vi "Test SLL DVR API Generator.vi"(6 "DVR API Suffix":string=" API", 8 "error in (no error)":errorcluster, 9 "DVR API Directory Path":path=path "D:/GitHub/LabVIEW/SLL/Tools/Class DVR API Generator/Example/APIs", 10 "Class Method Directory":path=path "D:/GitHub/LabVIEW/SLL/Tools/Class DVR API Generator/Example/Methods", 11 "Class Path":path=path "D:/GitHub/LabVIEW/SLL/Tools/Class DVR API Generator/Example/My Sample Class.lvclass") -> (0 "error out":errorcluster)   [LabVIEW 2016, in "SLL Scripting.lvlib"]
uses:
  SLL Scripting.lvlib
  SLL Class DVR API Generator.lvlib
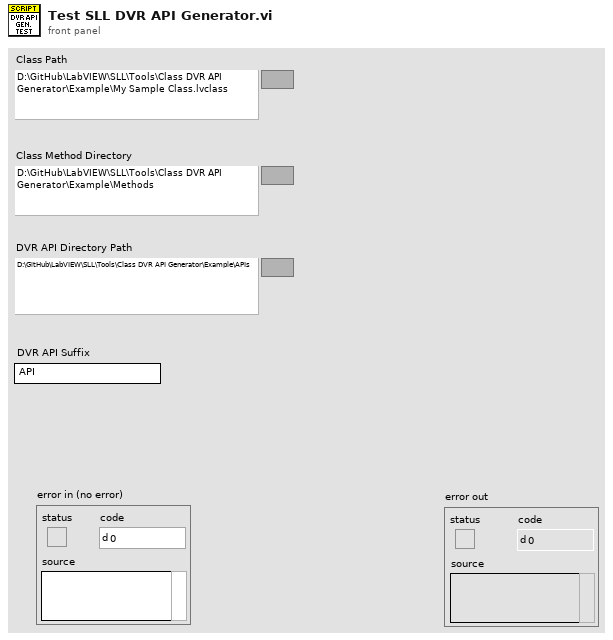
[diagram p1: front panel]
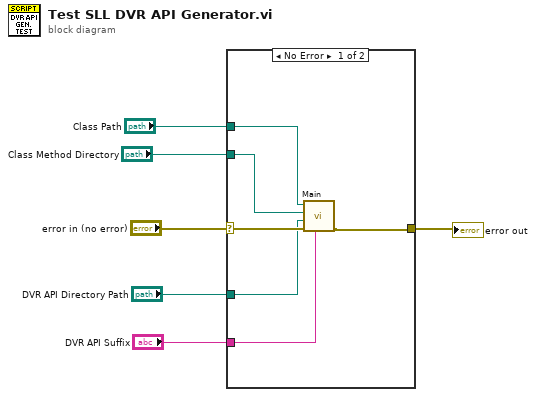
[diagram p0: block diagram]
diagram:
  n1 = case shown="No Error" "error in (no error)" {
    selector: "error in (no error)" -> [w12 w13]
    tunnel: [w11 w13] -> w5
    tunnel: "Class Path" -> [w10 _]
    tunnel: "DVR API Suffix" -> [w7 _]
    tunnel: "Class Method Directory" -> [w9 _]
    tunnel: "DVR API Directory Path" -> [w8 _]
    frame No Error {
      n2 = call "Main.vi"("DVR API Suffix"=w7, "error in (no error)"=w12, "DVR API Directory Path"=w8, "Class Method Directory"=w9, "Class Path"=w10) -> ("error out"=w11:errorcluster)  [unwired: 6 in]
    }
    frame Error {
    }
  }
  "error out" <- w5
